vi "ModifyTableEntry.vi"(8 "error in (no error)":errorcluster, 11 "HealthCheck in":refnum<class "HealthCheck.lvclass">) -> (0 "error out":errorcluster, 3 "HealthCheck out":refnum<class "HealthCheck.lvclass">)   [LabVIEW 2018, in "HealthCheck.lvclass"]
uses:
  HealthCheck.lvclass
  DataEntry_TypeDef.ctl
  HealthCheck.lvclass/HealthCheck.ctl
panel:
  in  "Cancel":bool
  in  "Save":bool
  in  "Table Control":string[][](table)=[["Right linear hall effect", "cm", "0", "", "5", "1"], ["Left linear hall effect", "cm", "0", "", "5", "1"], ["24V  battery voltage", "V", "24", "", "29", "1"], ["24V battery current", "A", "0", "", "20", "1"], ["24V battery temp", "C", "0", "", "50", "1"], ["BMS1 pack voltage", "V", "186", "", "252", "0"], ["BMS1 pack current", "A", "0", "", "400", "0"], ["BMS1 max temp", "F", "0", "", "80", "1"], ["BMS2 pack voltage", "V", "148.8", "", "201.6", "1"], ["BMS2 pack current", "A", "0", "", "400", "0"], ["BMS2 max temp", "F", "0", "", "80", "1"], ["Motor temp", "C", "0", "", "120", "1"], ["motor-controller temp", "C", "0", "", "60", "1"], ["Tank PT", "psig", "0", "", "3000", "0"], ["Pump PT", "psig", "15", "", "99999", "0"], ["Brake PT", "psig", "0", "", "150", "1"], ["IMU acceleration", "g", "-2.1", "", "0.716", "2"], ["PV1 pressure", "psig", "15", "", "30", "1"], ["PV2 pressure", "psig", "15", "", "30", "1"]]
  # "While VI is NOT running, permanently save changes by:\n• right click the table\n• select \"Data Operations\"  -> \"Make Current Value Default\"\n• save the VI"
  # "Optional, hide these from user"
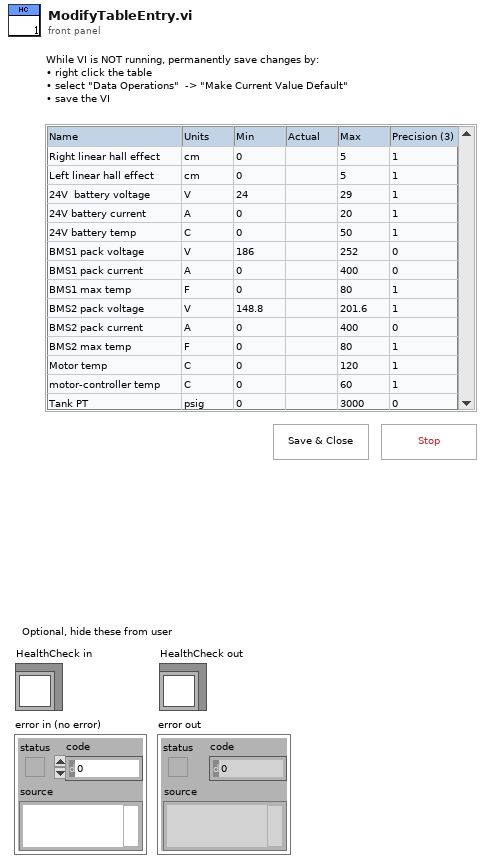
[diagram p1: front panel]
types:
  T1 = typedef "HealthCheck.lvclass/DataEntry_TypeDef.ctl" = cluster{"Data Name":string, "Units":string, "Minimum Value":string, "Maximum Value":string, "Actual Value":string, "Precision":i16}
  T2 = enum32{"Invalid", "Standard", "Closed", "Hidden", "Minimized", "Maximized"}
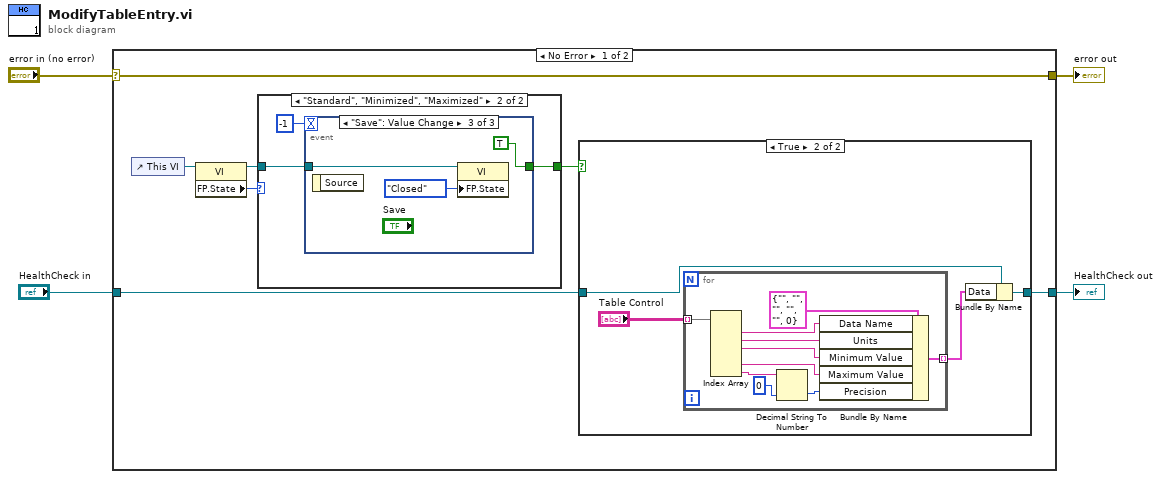
[diagram p0: block diagram]
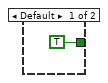
[diagram p3: hidden frame]
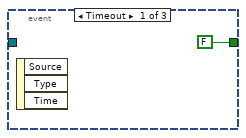
[diagram p4: hidden frame]
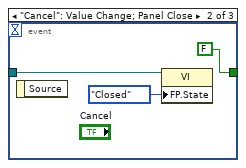
[diagram p5: hidden frame]
diagram:
  n1 = case shown="No Error" "error in (no error)" {
    selector: "error in (no error)" -> [w11 w39]
    tunnel: [w11 w39] -> w3
    tunnel: [w10 w38] -> w1
    tunnel: "HealthCheck in" -> [w9 w38]
    frame No Error {
      n2 = control-ref of="This VI"() -> (w7:refnum<vi>)
      n3 = property class="VI"(reference=w7) -> (reference out=w5:refnum<vi>, "FP.State"=w8:T2)  [unwired: 1 in, 1 out]
      n4 = case shown="\"Standard\", \"Minimized\", \"Maximized\"" w8 {
        tunnel: [TRUE ("Cancel") w29] -> w6
        tunnel: w5 -> [_ w28]
        frame Default {
        }
        frame "Standard", "Minimized", "Maximized" {
          n5 = event shown="[2] \"Save\": Value Change" {
            selector: _ -> [_ _ _]
            dyn-events: _ -> [_ _ _]
            timeout: -1 -> [_ _ _]
            tunnel: [FALSE ("Cancel") FALSE ("Cancel") TRUE ("Cancel")] -> w29
            tunnel: w28 -> [_ w33 w35]
            event Timeout {
              n6 = event-data() -> ()  [unwired: 1 in, 3 out]
            }
            event "Cancel": Value Change; Panel Close {
              n7 = event-data() -> ()  [unwired: 1 in, 1 out]
              n8 = property class="VI"(reference=w33, "FP.State"=T2."Closed" ("Front Panel Window:State")) -> ()  [unwired: 1 in, 2 out]
            }
            event "Save": Value Change {
              n9 = event-data() -> ()  [unwired: 1 in, 1 out]
              n10 = property class="VI"(reference=w35, "FP.State"=T2."Closed" ("Front Panel Window:State")) -> ()  [unwired: 1 in, 2 out]
            }
          }
        }
      }
      n11 = case shown="True" w6 {
        tunnel: [w12 w15] -> w10
        tunnel: w9 -> [w12 w14]
        frame False {
        }
        frame True {
          n12 = for {
            tunnel: "Table Control" -> [w26] mode=indexing
            tunnel: [w24] -> w13 mode=indexing
            n13 = Index Array(array=w26) -> (element #1=w23:string, element #2=w22:string, element #3=w21:string, element #5=w20:string, element #6=w19:string)  [unwired: 6 in, 1 out]
            n14 = Decimal String To Number(string=w19, default (0L)=i16 0 ("default (0 I32)")) -> (number=w18:i16)  [unwired: 1 in, 1 out]
            n15 = Bundle By Name(cluster=T1 {"Data Name"="", "Units"="", "Minimum Value"="", "Maximum Value"="", "Actual Value"="", "Precision"=0} ("Sensor Info"), "Data Name"=w23, "Units"=w22, "Minimum Value"=w21, "Maximum Value"=w20, "Precision"=w18) -> (w24:T1)
          }
          n16 = Bundle By Name(cluster=w14, "Data"=w13) -> (w15:refnum<class "HealthCheck.lvclass">)
        }
      }
    }
    frame Error {
    }
  }
  "error out" <- w3
  "HealthCheck out" <- w1
